vi "Untitled 1.vi"() -> ()   [LabVIEW 2016]
panel:
  in  "stop":bool
  out "number (0 to 1)":dbl
  out "i":i32
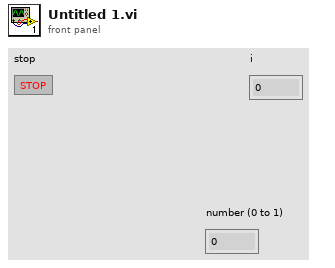
[diagram p1: front panel]
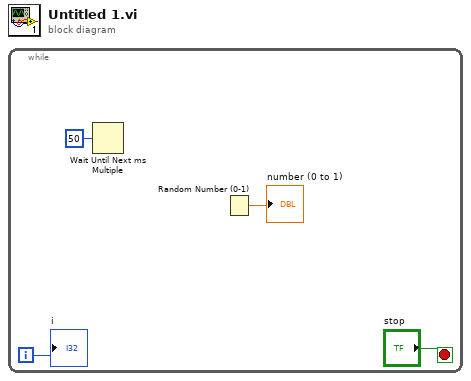
[diagram p0: block diagram]
diagram:
  n1 = while {
    i -> [w4]
    stop <- "stop" stop-if-true
    n2 = Wait Until Next ms Multiple(millisecond multiple=u32 50) -> ()  [unwired: 1 out]
    n3 = Random Number (0-1)() -> (number: 0 to 1=→"number (0 to 1)":dbl)
    "i" <- w4
  }
